vi "Laurel Buffer Reset.vi"(8 "error in (no error)":errorcluster, 11 "VISA Refnum in":refnum<visa-resource-name>) -> (0 "error out":errorcluster, 3 "VISA Refnum out":refnum<visa-resource-name>)   [LabVIEW 2023]
uses:
  <vilib>/Instr/_visa.llb/VISA Open Access Mode.ctl
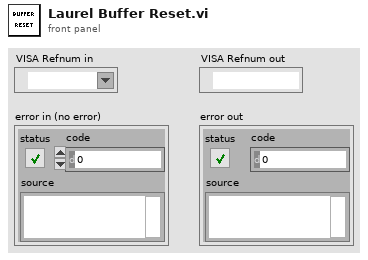
[diagram p1: front panel]
types:
  T1 = typedef "VISA Open Access Mode.ctl" = u32
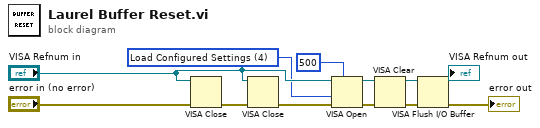
[diagram p0: block diagram]
diagram:
  w8 = T1 4 items=["VISA Defaults"=0, "Exclusive Lock"=1, "Load Configured Settings"=4] ("Access Mode")
  n1 = VISA Close(VISA resource name="VISA Refnum in", error in (no error)="error in (no error)") -> (error out=w6:errorcluster)
  n2 = VISA Close(VISA resource name="VISA Refnum in", error in (no error)=w6) -> (error out=w7:errorcluster)
  n3 = VISA Open(timeout (0)=u32 500 ("VISA Open timeout (0)"), access mode=w8, error in (no error)=w7, VISA resource name="VISA Refnum in") -> (VISA resource name=w12:refnum<visa-resource-name>, error out=w10:errorcluster)  [unwired: 1 in]
  n4 = VISA Clear(VISA resource name=w12, error in (no error)=w10) -> (VISA resource name out=w1:refnum<visa-resource-name>, error out=w3:errorcluster)
  n5 = VISA Flush I/O Buffer(VISA resource name=w1, error in (no error)=w3) -> (VISA resource name out=→"VISA Refnum out":refnum<visa-resource-name>, error out=→"error out":errorcluster)  [unwired: 1 in]
